vi "Rectangle.vi"(8 "error in (no error)":errorcluster, 10 "target":refnum<class "pRectangle.lvclass">, 11 "pRectangle in":refnum<class "pRectangle.lvclass">) -> (0 "error out":errorcluster, 3 "pRectangle out":refnum<class "pRectangle.lvclass">)   [LabVIEW 2017, in "pRectangle.lvclass"]
uses:
  pRectangle.lvclass
  C:/Users/fflores/Documents/LabVIEW-Open-Projects/LabIVEW OOP Design Patterns/Prototype Pattern/Shape Class/pShape.lvclass
  pRectangle.lvclass/pRectangle.ctl
  Shape Class/pShape.lvclass
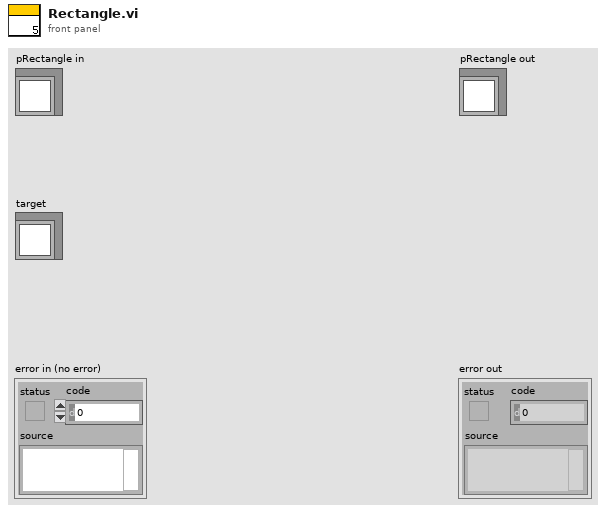
[diagram p1: front panel]
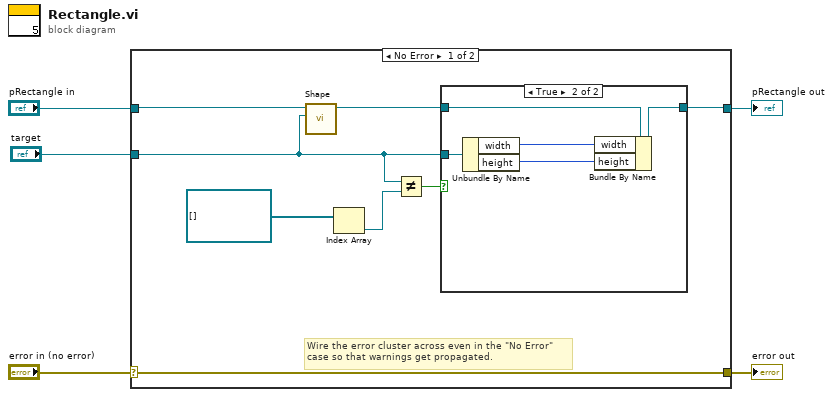
[diagram p0: block diagram]
diagram:
  n1 = case shown="No Error" "error in (no error)" {
    selector: "error in (no error)" -> [w13 w21]
    tunnel: [w13 w21] -> w4
    tunnel: [w8 w20] -> w2
    tunnel: "pRectangle in" -> [w7 w20]
    tunnel: "target" -> [w6 _]
    frame No Error {
      # "Wire the error cluster across even in the \"No Error\"\ncase so that warnings get propagated."
      n2 = call "Shape.vi"("pShape.lvclass"=w6, "pShape in"=w7) -> ("pShape out"=w10:refnum<class "pRectangle.lvclass">)  [unwired: 8 in, 1 out]
      n3 = Index Array(array=refnum<class "pRectangle.lvclass">[] []) -> (element=w12:refnum<class "pRectangle.lvclass">)  [unwired: 1 in]
      n4 = Not Equal?(x=w6, y=w12) -> (x != y?=w9:bool)
      n5 = case shown="True" w9 {
        tunnel: [w14 w18] -> w8
        tunnel: w10 -> [w14 w19]
        tunnel: w6 -> [_ w17]
        frame False {
        }
        frame True {
          n6 = Unbundle By Name(w17) -> ("width"=w16:i32, "height"=w15:i32)
          n7 = Bundle By Name(cluster=w19, "width"=w16, "height"=w15) -> (w18:refnum<class "pRectangle.lvclass">)
        }
      }
    }
    frame Error {
    }
  }
  "error out" <- w4
  "pRectangle out" <- w2
